vi "Enforcer.vi"(8 "error in (no error)":errorcluster, 11 "Path":path) -> (0 "error out":errorcluster, 3 "dup Folder Path":path)   [LabVIEW 2016]
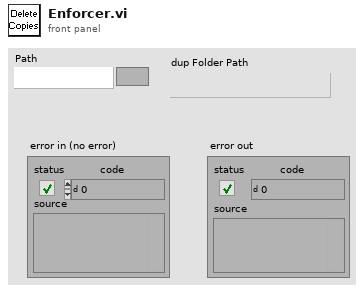
[diagram p1: front panel]
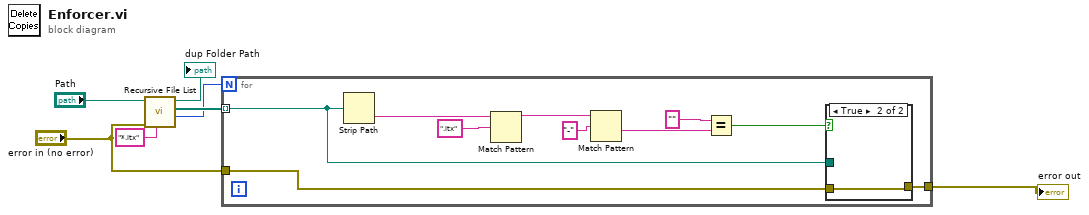
[diagram p0: block diagram]
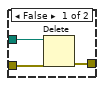
[diagram p2: hidden frame]
diagram:
  n1 = call <vilib>:"Recursive File List.vi"("pattern"="*.itx", "error in (no error)"="error in (no error)", "Folder Path"="Path") -> ("Number of Files"=w5:i32, "All Files in Dir"=w6:path[], "dup Folder Path"=→"dup Folder Path":path)  [unwired: 5 in, 1 out]
  n2 = for {
    N: w5 -> [_]
    tunnel: w6 -> [w10] mode=indexing
    tunnel: [w9] -> w3
    tunnel: "error in (no error)" -> [w8]
    n3 = Strip Path(path=w10) -> (name=w17:string)  [unwired: 1 out]
    n4 = Match Pattern(string=w17, regular expression=".itx") -> (before substring=w15:string)  [unwired: 1 in, 3 out]
    n5 = Match Pattern(string=w15, regular expression="-") -> (after substring=w13:string)  [unwired: 1 in, 3 out]
    n6 = Equal?(x="", y=w13) -> (x = y?=w11:bool)
    n7 = case shown="True" w11 {
      tunnel: w10 -> [w20 _]
      tunnel: [w19 w21] -> w9
      tunnel: w8 -> [w18 w21]
      frame False {
        n8 = Delete(path (use dialog)=w20, error in=w18) -> (error out=w19:errorcluster)  [unwired: 3 in, 2 out]
      }
      frame True {
      }
    }
  }
  "error out" <- w3
